vi "svc_Complex to Mag2 Array.vi"(4 "complex array":cdb[](array[numeric]) format="%.2f") -> (1 "magnitude^2 array":dbl[](array[numeric]) format="%.2f")   [LabVIEW 2017]
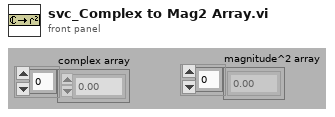
[diagram p1: front panel]
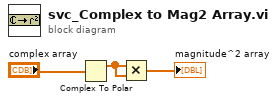
[diagram p0: block diagram]
diagram:
  n1 = Complex To Polar(r * e^(i*theta)="complex array") -> (r=w3:dbl[])  [unwired: 1 out]
  n2 = Multiply(x=w3, y=w3) -> (x*y=→"magnitude^2 array":dbl[])
